vi "XNET IP Stack Clear.vi"(0 "stack":refnum<k21>, 11 "error in":errorcluster) -> (15 "error out":errorcluster)   [LabVIEW 2018]
doc: "Clears (closes) the XNET IP Stack."
uses:
  nixlvapi.dll
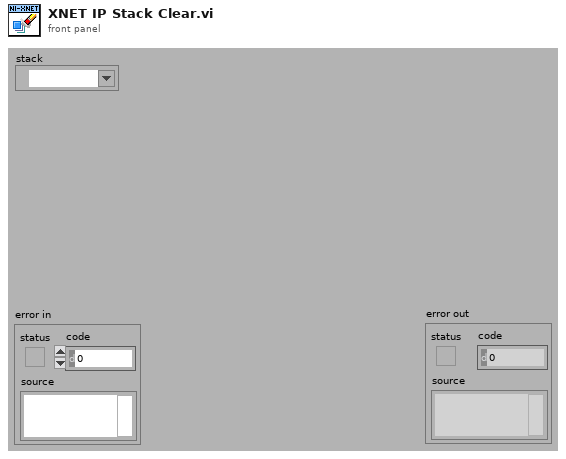
[diagram p1: front panel]
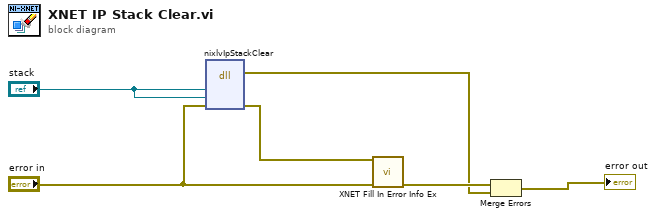
[diagram p0: block diagram]
diagram:
  n1 = dll-call lib="nixlvapi.*" fn="nixlvIpStackClear" label="Call Library"("reference"="stack", "refObjPtr"="stack", "errorInOut"="error in") -> (error out=w1:errorcluster, "errorInOut"=w6:errorcluster)  [unwired: 3 in, 4 out]
  n2 = call "XNET Fill In Error Info Ex.vi"("error xnet"=w6, "error in"="error in") -> ("error out"=w2:errorcluster)  [unwired: 13 in]
  n3 = Merge Errors(w2, w1) -> (→"error out":errorcluster)
